vi "run_main_panel.vi"(6 "Break Button":refnum<vi>, 8 "Stop Button":refnum<vi>, 9 "Pause Button":refnum<vi>, 10 "Reset":refnum<vi>, 11 "Run":refnum<vi>) -> ()   [LabVIEW 2019]
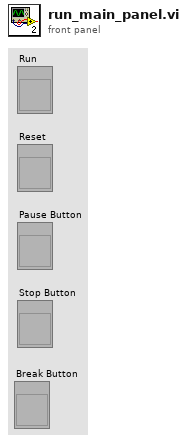
[diagram p1: front panel]
types:
  T1 = enum8{"Enabled", "Disabled", "Disabled and Grayed Out"}
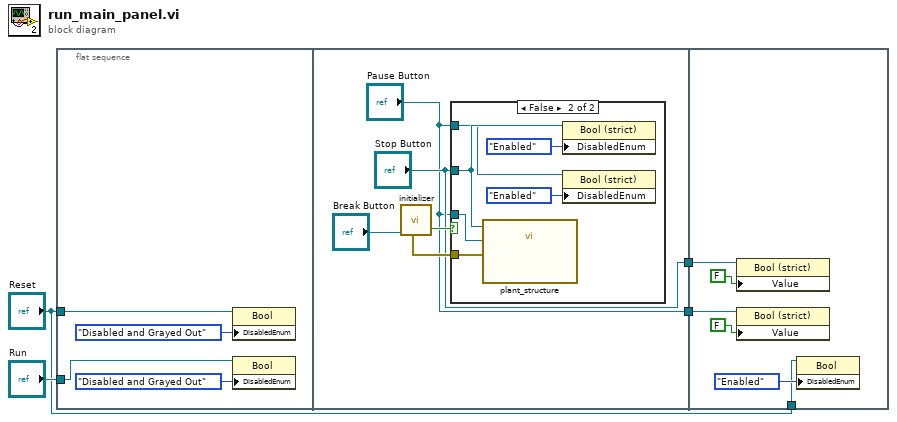
[diagram p0: block diagram]
diagram:
  n1 = flat-sequence {
    tunnel: "Run" -> [w6]
    tunnel: "Reset" -> [w5]
    tunnel: ["Stop Button"] -> w2
    tunnel: ["Pause Button"] -> w1
    tunnel: "Reset" -> [w23]
    tunnel: w2 -> [w21]
    tunnel: w1 -> [w20]
    frame #0 {
      n2 = property on="Property Node" class="Bool"(reference=w5, "DisabledEnum"=T1."Disabled and Grayed Out" ("Disabled")) -> ()  [unwired: 1 in, 2 out]
      n3 = property on="Property Node" class="Bool"(reference=w6, "DisabledEnum"=T1."Disabled and Grayed Out" ("Disabled")) -> ()  [unwired: 1 in, 2 out]
    }
    frame #1 {
      n4 = call "initializer.vi"("Break"="Break Button") -> ("Cancelled?"=w12:bool, "Dataflow Out"=w13:errorcluster)  [unwired: 5 in]
      n5 = case shown="False" w12 {
        tunnel: w13 -> [_ w17]
        tunnel: "Pause Button" -> [_ w16]
        tunnel: "Stop Button" -> [_ w15]
        tunnel: "Pause Button" -> [_ w14]
        frame True {
        }
        frame False {
          n6 = call "plant_structure.vi"("Dataflow"=w17, "Pause"=w16, "Stop"=w15) -> ()  [unwired: 9 in]
          n7 = property on="Property Node" class="Bool (strict)"(reference=w15, "DisabledEnum"=T1."Enabled" ("Disabled")) -> ()  [unwired: 1 in, 2 out]
          n8 = property on="Property Node" class="Bool (strict)"(reference=w14, "DisabledEnum"=T1."Enabled" ("Disabled")) -> ()  [unwired: 1 in, 2 out]
        }
      }
    }
    frame #2 {
      n9 = property on="Property Node" class="Bool (strict)"(reference=w21, "Value"=FALSE) -> ()  [unwired: 1 in, 2 out]
      n10 = property on="Property Node" class="Bool (strict)"(reference=w20, "Value"=FALSE ("Stop Button")) -> ()  [unwired: 1 in, 2 out]
      n11 = property on="Property Node" class="Bool"(reference=w23, "DisabledEnum"=T1."Enabled" ("Disabled")) -> ()  [unwired: 1 in, 2 out]
    }
  }
